vi "SetMoveParameters.vi"(8 "error in (no error)":errorcluster, 10 "Jog Parameters":T1, 11 "TranslationStageUI.lvclass":refnum<class "TranslationStageUI.lvclass">) -> (0 "error out":errorcluster, 3 "TranslationStageUI.lvclass":refnum<class "TranslationStageUI.lvclass">)   [LabVIEW 2023]
uses:
  TranslationStageUI.lvclass
  C:/Program Files/National Instruments/LabVIEW 2023/vi.lib/ActorFramework/Actor/Actor.lvclass
  C:/Users/quantum/Documents/LVDAQ/UIs/TranslationStage_UI/TranslationStage_UI/TranslationStageUI.lvclass
  C:/Users/quantum/Documents/LVDAQ/Interfaces/InitDeinitInterface/InitDeinitComm/InitDeinitComm.lvclass
  C:/Users/quantum/Documents/LVDAQ/Interfaces/AbstractInstrumentClasses/TranslationStages_LV/TranslationStagesComm/TranslationStagesComm.lvclass
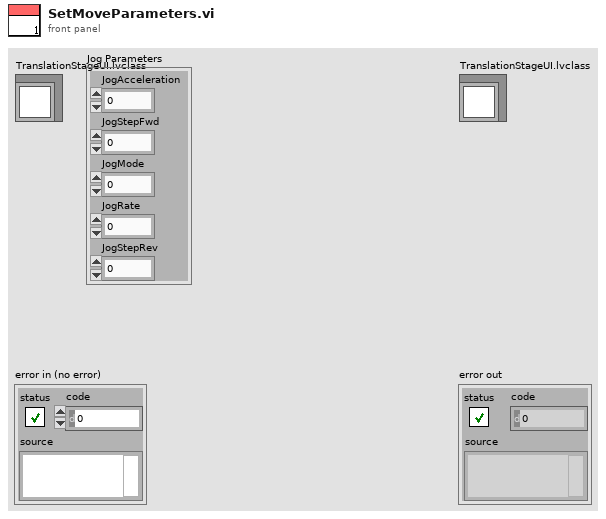
[diagram p1: front panel]
types:
  T1 = cluster{"JogAcceleration":i32, "JogStepFwd":i32, "JogMode":i32, "JogRate":i32, "JogStepRev":i32}
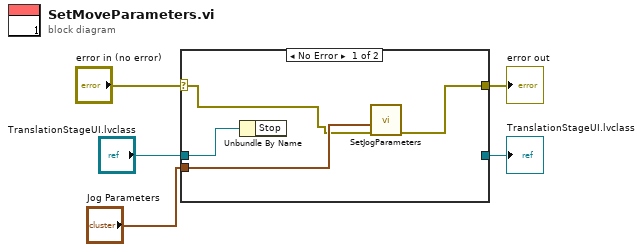
[diagram p0: block diagram]
diagram:
  n1 = case shown="No Error" "error in (no error)" {
    selector: "error in (no error)" -> [w6 w11]
    tunnel: [w7 w11] -> w4
    tunnel: [_ w10] -> w2
    tunnel: "TranslationStageUI.lvclass" -> [w9 w10]
    tunnel: "Jog Parameters" -> [w8 _]
    frame No Error {
      n2 = Unbundle By Name(w9) -> ()  [unwired: 1 out]
      n3 = call "SetJogParameters.vi"("error in (no error)"=w6, "Jog Parameters"=w8) -> ("error out"=w7:errorcluster)  [unwired: 8 in, 1 out]
    }
    frame Error {
    }
  }
  "error out" <- w4
  "TranslationStageUI.lvclass" <- w2
